vi "Сканер.vi"() -> ()   [LabVIEW 2016]
uses:
  GlobalVariable.vi
  <vilib>/Instr/_visa.llb/VISA Configure Serial Port (Instr).vi
panel:
  out "ReadNumber":i32
  out "Gauge":cluster{dbl, dbl}(knob) scale=0.0..360.0
  out "ScrollPosBool":bool
  out "Serial Settings:Number of Bytes at Serial Port":u32
  in  "XON/XOFF Символ":cluster{"XON":u8, "XOFF":u8}={"XON"=17, "XOFF"=19} {"XOFF" items=["NUL", "SOH", "STX", "ETX", "EOT", "ENQ", "ACK", "BEL", "BS", "HT", "LF", "VT", "FF", "CR", "SO", "SI", "DLE", "DC1", "DC2", "DC3", "DC4", "NAK", "SYN", "ETB", "CAN", "EM", "SUB", "ESC", "FS", "GS", "RS", "US", "SP", "!", "\"", "#", "$", "%", "&", "'", "(", ")", "*", "+", ",", "- (-)", ".", "/", "0", "1", "2", "3", "4", "5", "6", "7", "8", "9", ":", ";", "<", "=", ">", "?", "@", "A", "B", "C", "D", "E", "F", "G", "H", "I", "J", "K", "L", "M", "N", "O", "P", "Q", "R", "S", "T", "U", "V", "W", "X", "Y", "Z", "[", "\\", "]", "^", "_", "`", "a", "b", "c", "d", "e", "f", "g", "h", "i", "j", "k", "l", "m", "n", "o", "p", "q", "r", "s", "t", "u", "v", "w", "x", "y", "z", "{", "|", "}", "~"]; "XON" items=["NUL", "SOH", "STX", "ETX", "EOT", "ENQ", "ACK", "BEL", "BS", "HT", "LF", "VT", "FF", "CR", "SO", "SI", "DLE", "DC1", "DC2", "DC3", "DC4", "NAK", "SYN", "ETB", "CAN", "EM", "SUB", "ESC", "FS", "GS", "RS", "US", "SP", "!", "\"", "#", "$", "%", "&", "'", "(", ")", "*", "+", ",", "- (-)", ".", "/", "0", "1", "2", "3", "4", "5", "6", "7", "8", "9", ":", ";", "<", "=", ">", "?", "@", "A", "B", "C", "D", "E", "F", "G", "H", "I", "J", "K", "L", "M", "N", "O", "P", "Q", "R", "S", "T", "U", "V", "W", "X", "Y", "Z", "[", "\\", "]", "^", "_", "`", "a", "b", "c", "d", "e", "f", "g", "h", "i", "j", "k", "l", "m", "n", "o", "p", "q", "r", "s", "t", "u", "v", "w", "x", "y", "z", "{", "|", "}", "~"]}
  in  "Ошибка порта":T1
  in  "Номер COM порта":refnum<visa-resource-name>
  in  "Clear":bool
  in  "ReadStringON":bool
  in  "WriteStringON":bool
  in  "В конце записи добавить идентификатор завершения":bool=TRUE
  out "IndStartStop":bool
  in  "Exit":bool
  in  "Start":bool
  in  "Stop":bool
  out "Return Count Read":u32
  in  "В конце чтения добавить идентификатор завершения":bool=TRUE
  in  "Идентификатор завершения":u8=10 format="%.0x"
  out "Read String":string
  out "Return Count Write":u32
  in  "Write String":string="*IDN?"
  in  "Параметры порта":T2={"Бит в секунду: "=9600, "Биты данных:"=8, "Чётность"=0, "Стоповые биты"=10, "Управление потоком"=0} {"Управление потоком" items=["Нет"=0, "Xon/Xoff"=1, "RTS/CTS"=2, "DTR/DSR"=4]; "Стоповые биты" items=["1.0"=10, "1.5"=15, "2.0"=20]; "Чётность" items=["Нет", "Нечётный", "Чётный", "Маркер", "Пробел"]; "Биты данных:" items=["4"=4, "5"=5, "6"=6, "7"=7, "8"=8]; "Бит в секунду:" items=["75"=75, "110"=110, "134"=134, "150"=150, "300"=300, "600"=600, "1200"=1200, "1800"=1800, "2400"=2400, "4800"=4800, "7200"=7200, "9600"=9600, "14400"=14400, "19200"=19200, "28800"=28800, "38400"=38400, "56000"=56000, "57600"=57600, "115200"=115200, "128000"=128000, "230400"=230400]}
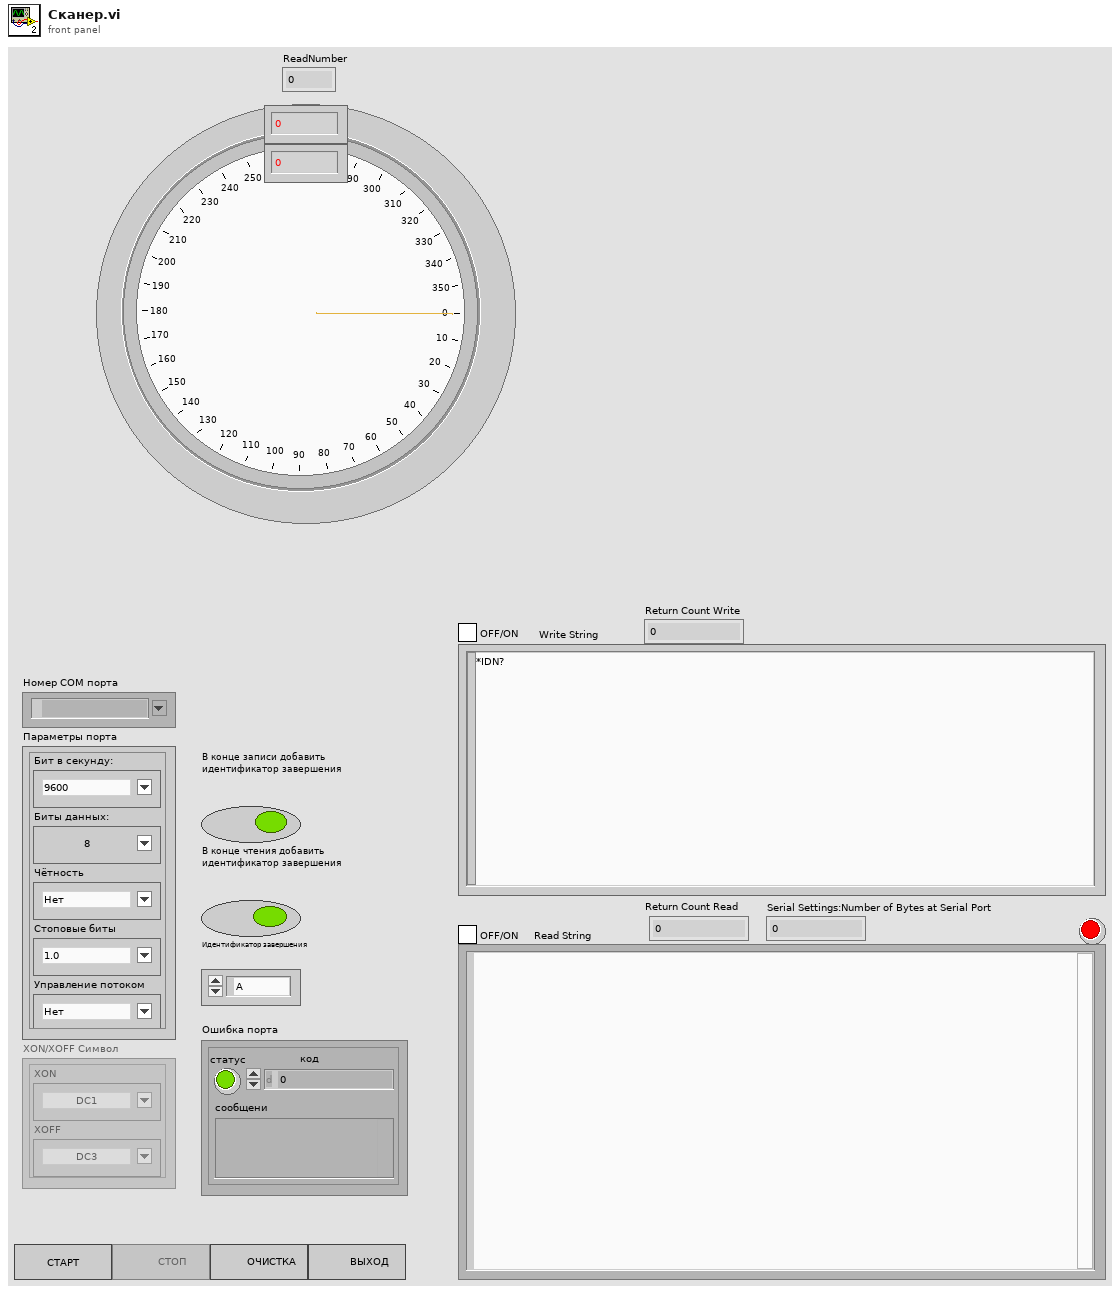
[diagram p1: front panel]
types:
  T1 = cluster{"статус":bool, "код":i32, "сообщени":string}
  T2 = cluster{"Бит в секунду: ":u32, "Биты данных:":u16, "Чётность":u16, "Стоповые биты":u16, "Управление потоком":u16}
  T3 = enum8{"Enabled", "Disabled", "Disabled and Grayed Out"}
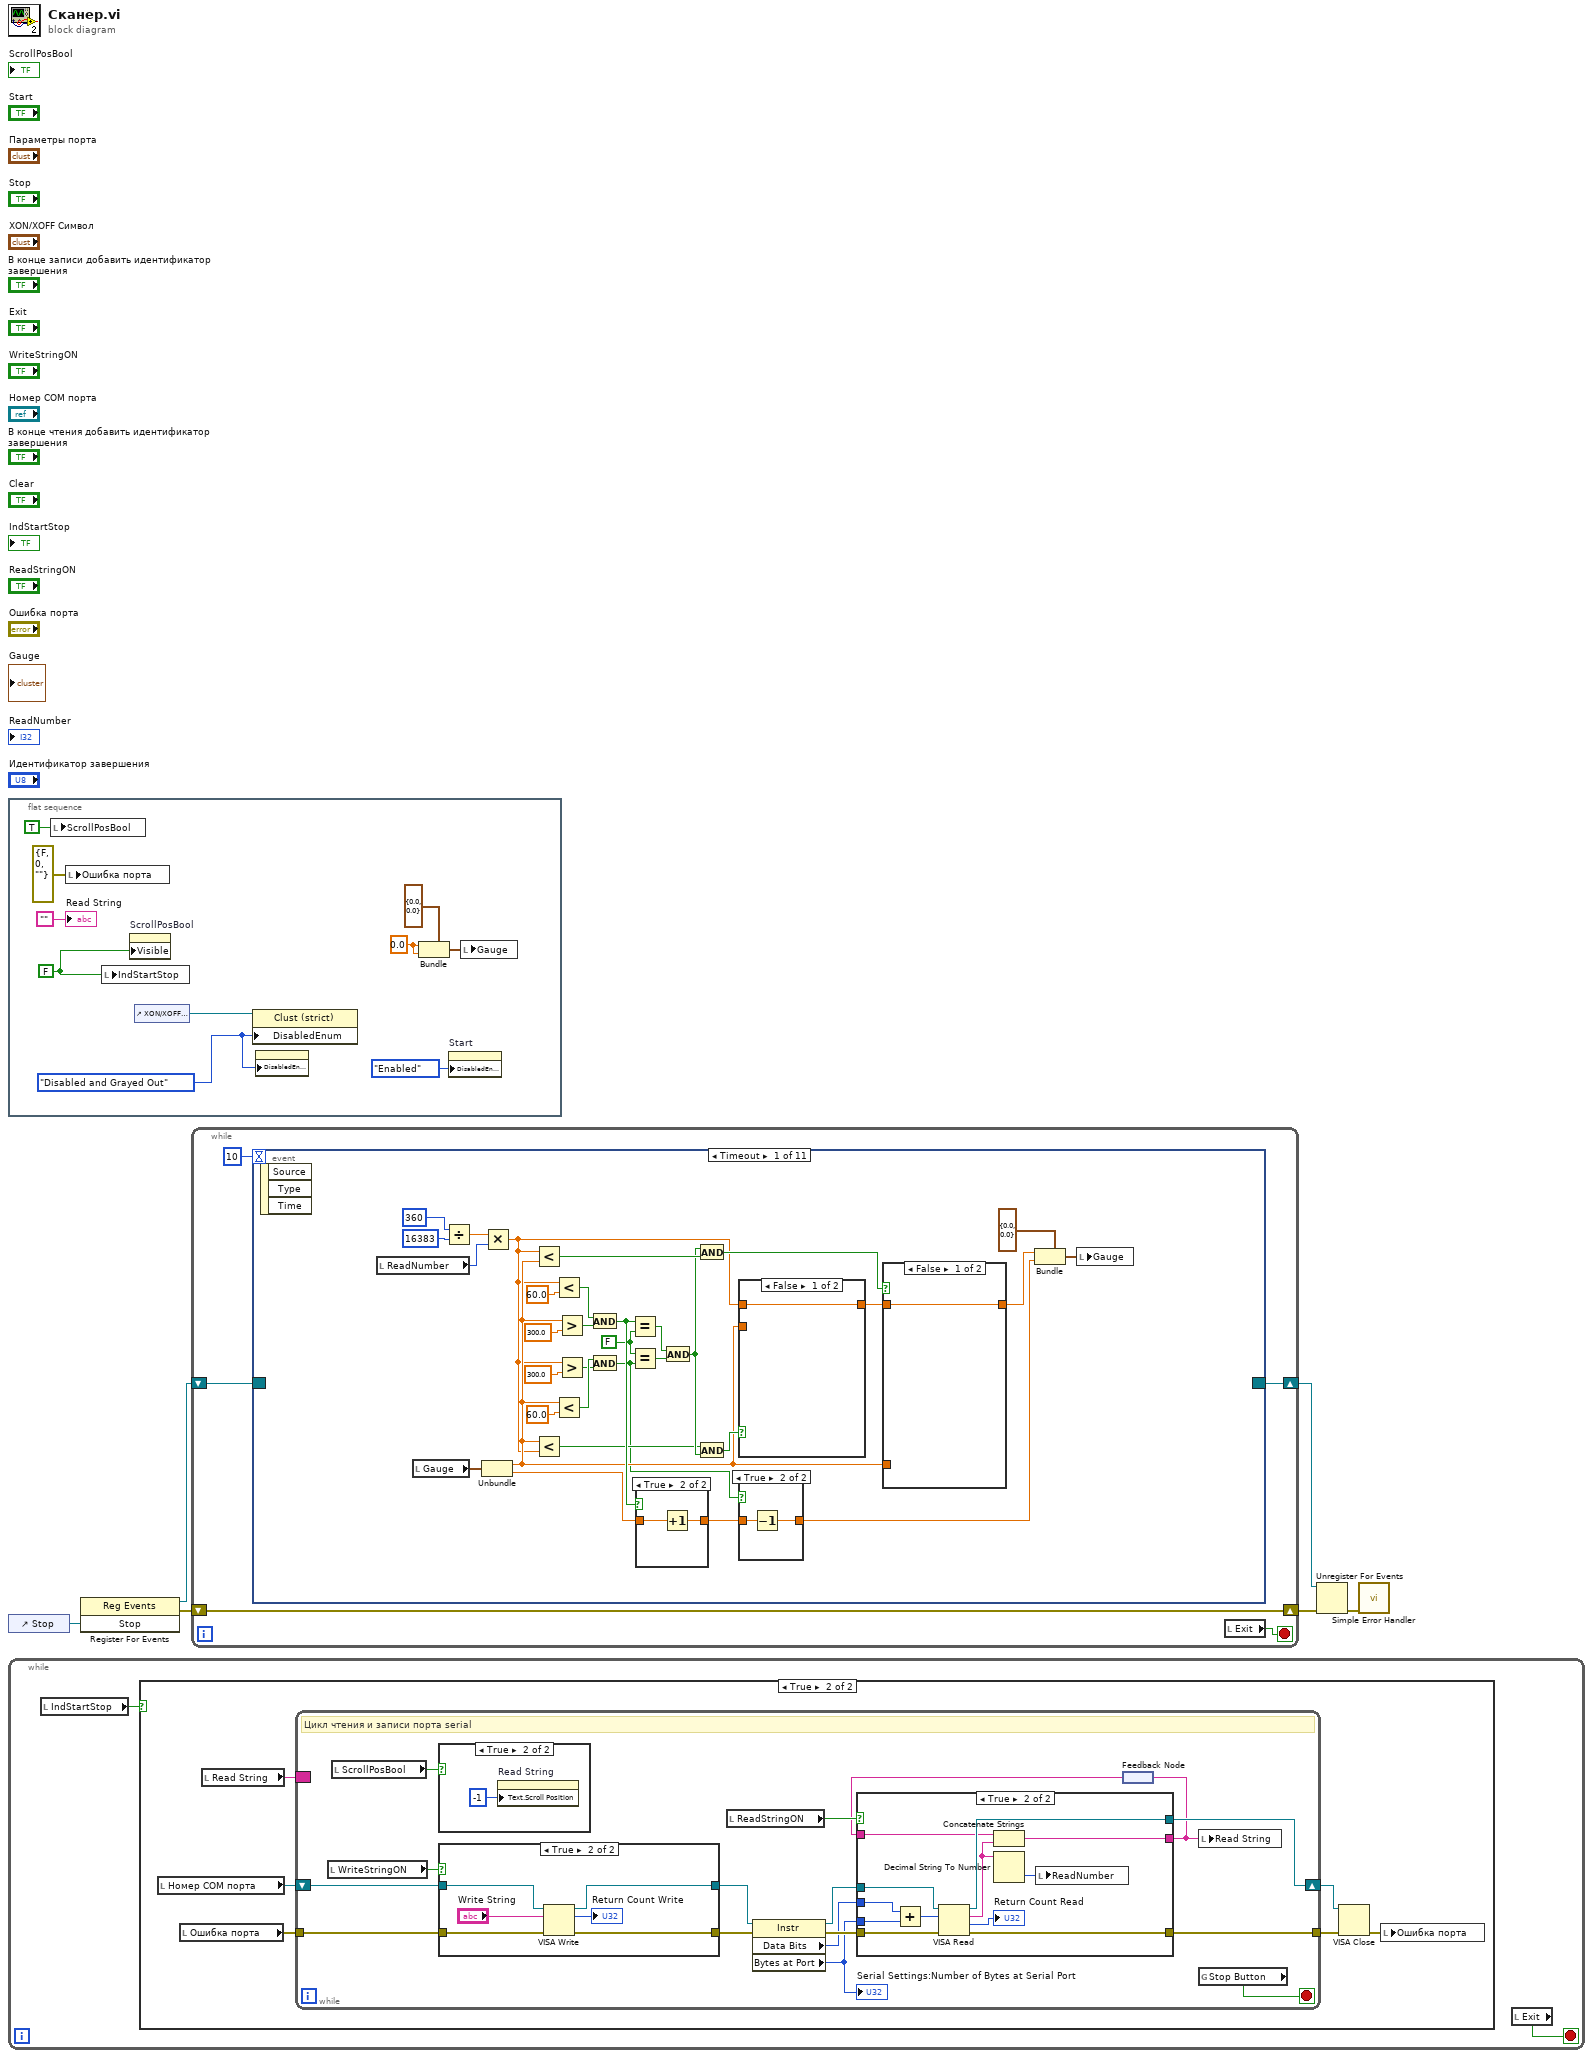
[diagram p0: block diagram]
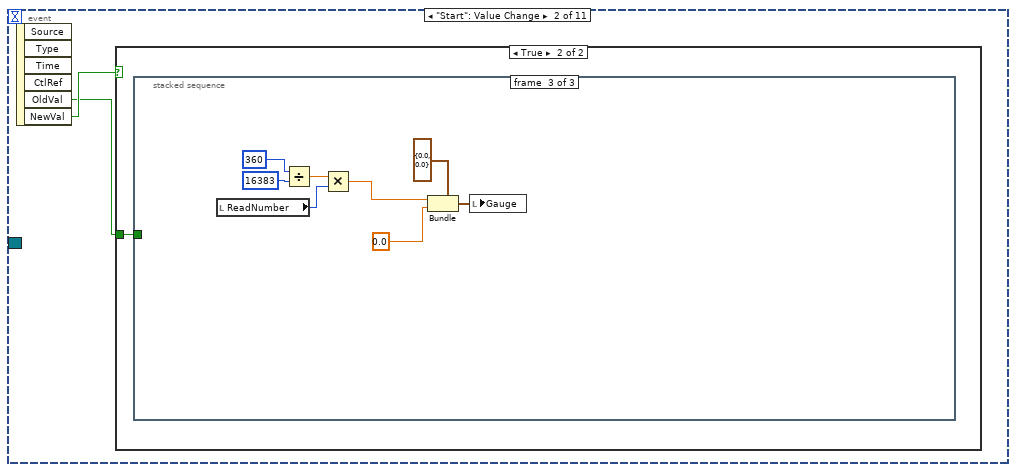
[diagram p10: hidden frame]
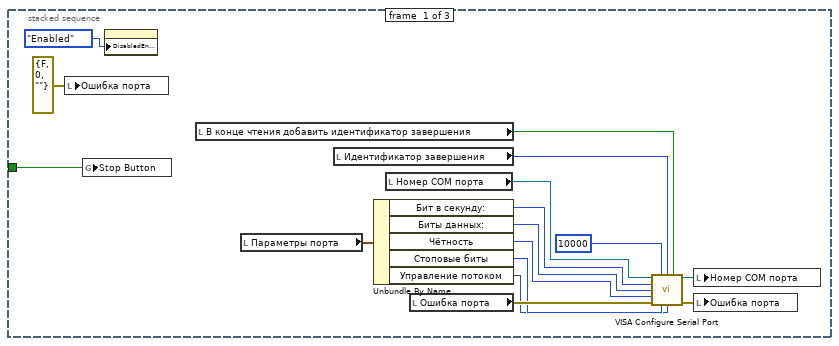
[diagram p12: hidden frame]
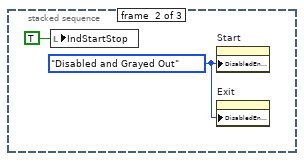
[diagram p13: hidden frame]
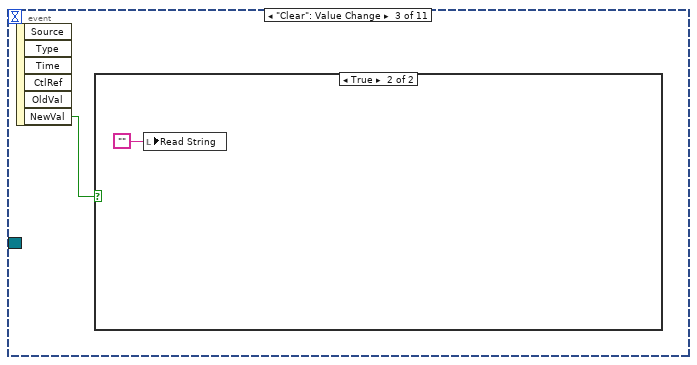
[diagram p14: hidden frame]
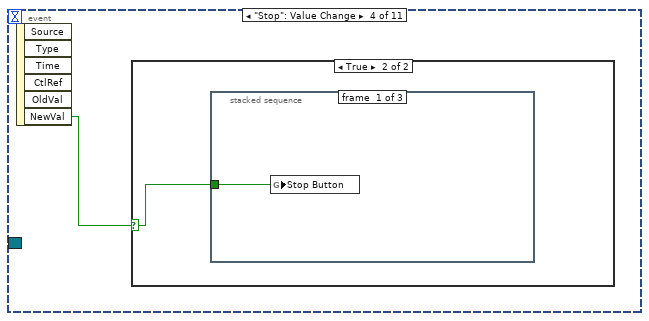
[diagram p16: hidden frame]
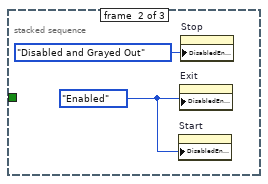
[diagram p18: hidden frame]
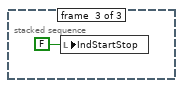
[diagram p19: hidden frame]
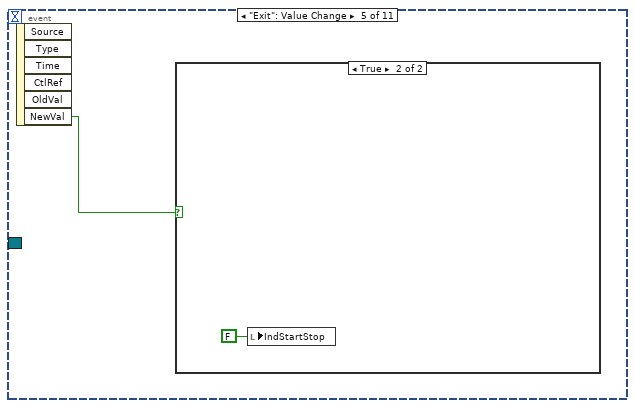
[diagram p20: hidden frame]
diagram:
  n1 = flat-sequence {
    frame #0 {
      w7 = 0.0
      w12 = FALSE
      w11 = T3."Disabled and Grayed Out" ("Disabled")
      n2 = local write "ScrollPosBool"(TRUE ("ScrollPosBool")) -> ()
      n3 = local write "Ошибка порта"(errorcluster {"status"=FALSE, "code"=0, "source"=""} ("error in (no error)")) -> ()
      n4 = local write "IndStartStop"(w12) -> ()
      n5 = property on="ScrollPosBool" class="Bool (strict)"("Visible"=w12) -> ()  [unwired: 2 in, 2 out]
      n6 = control-ref of="XON/XOFF Символ"() -> (w15:refnum<vi>)
      n7 = property class="Clust (strict)"(reference=w15, "DisabledEnum"=w11) -> ()  [unwired: 1 in, 2 out]
      n8 = property on="Stop" class="Bool (strict)"("DisabledEnum"=w11) -> ()  [unwired: 2 in, 2 out]
      n9 = Bundle(cluster=cluster{dbl, dbl} {0.0, 0.0} ("Gauge"), w7, w7) -> (w9:cluster{dbl, dbl})
      n10 = property on="Start" class="Bool (strict)"("DisabledEnum"=T3."Enabled" ("Disabled")) -> ()  [unwired: 2 in, 2 out]
      n11 = local write "Gauge"(w9) -> ()
      "Read String" <- ""
    }
  }
  n12 = control-ref of="Stop"() -> (w1:refnum<vi>)
  n13 = while {
    stop <- w17 stop-if-true
    n14 = local read "IndStartStop"() -> (w18:bool)
    n15 = case shown="True" w18 {
      frame False {
      }
      frame True {
        n16 = local read "Номер COM порта"() -> (w23:refnum<visa-resource-name>)
        n17 = local read "Ошибка порта"() -> (w24:T1)
        n18 = local read "Read String"() -> (w22:string)
        n19 = while {
          shift-right: [w31] -> w20
          shift-left: w23 -> [w32]
          tunnel: w24 -> [w33]
          tunnel: [w30] -> w19
          border: w22 -> [_]
          stop <- w27 stop-if-true
          # "Цикл чтения и записи порта serial"
          n20 = local read "WriteStringON"() -> (w36:bool)
          n21 = local read "ScrollPosBool"() -> (w34:bool)
          n22 = case shown="True" w34 {
            frame False {
            }
            frame True {
              n23 = property on="Read String" class="Str"("Text.Scroll Position"=-1) -> ()  [unwired: 2 in, 2 out]
            }
          }
          n24 = case shown="True" w36 {
            tunnel: [w58 w64] -> w40
            tunnel: [w57 w63] -> w39
            tunnel: w32 -> [w58 w62]
            tunnel: w33 -> [w57 w61]
            frame False {
            }
            frame True {
              n25 = VISA Write(VISA resource name=w62, write buffer="Write String", error in (no error)=w61) -> (VISA resource name out=w64:refnum<visa-resource-name>, return count=→"Return Count Write":u32, error out=w63:errorcluster)
            }
          }
          n26 = local read "ReadStringON"() -> (w35:bool)
          n27 = property class="Instr"(reference=w40, error in=w39) -> (reference out=w38:refnum<visa-resource-name>, error out=w37:errorcluster, "Data Bits"=w26:u16, "Bytes at Port"=w25:u32)
          "Serial Settings:Number of Bytes at Serial Port" <- w25
          n28 = feedback #1() -> (w29:string)
          n29 = case shown="True" w35 {
            tunnel: [w44 w56] -> w31
            tunnel: [w43 w52] -> w30
            tunnel: w25 -> [_ w51]
            tunnel: w38 -> [w44 w55]
            tunnel: w37 -> [w43 w54]
            tunnel: [w42 w49] -> w28
            tunnel: w29 -> [w42 w48]
            tunnel: w26 -> [_ w47]
            frame False {
            }
            frame True {
              n30 = Add(x=w47, y=w51) -> (x+y=w50:u32)
              n31 = VISA Read(VISA resource name=w55, byte count=w50, error in (no error)=w54) -> (VISA resource name out=w56:refnum<visa-resource-name>, read buffer=w46:string, return count=→"Return Count Read":u32, error out=w52:errorcluster)
              n32 = Concatenate Strings(w48, w46) -> (w49:string)
              n33 = Decimal String To Number(string=w46) -> (number=w45:i32)  [unwired: 2 in, 1 out]
              n34 = local write "ReadNumber"(w45) -> ()
            }
          }
          n35 = feedback-in #1(w28) -> ()
          n36 = local write "Read String"(w28) -> ()
          n37 = global read "GlobalVariable.vi" "Stop Button"() -> (w27:bool)
        }
        n38 = VISA Close(VISA resource name=w20, error in (no error)=w19) -> (error out=w21:errorcluster)
        n39 = local write "Ошибка порта"(w21) -> ()
      }
    }
    n40 = local read "Exit"() -> (w17:bool)
  }
  n41 = register-events(w1) -> (reference out=w6:refnum<event-registration>, error out=w5:errorcluster)  [unwired: 2 in]
  n42 = while {
    shift-right: [w67] -> w4
    shift-left: w6 -> [w68]
    shift-right: [w66] -> w3
    shift-left: w5 -> [w66]
    stop <- w65 stop-if-true
    n43 = event shown="[0] Timeout" {
      selector: w68 -> [_ _ _ _ _ _ _ _ _ _ _]
      dyn-events: [_ _ _ _ _ _ _ _ _ _ _] -> w67
      timeout: 10 -> [_ _ _ _ _ _ _ _ _ _ _]
      event Timeout {
        w72 = FALSE
        n44 = event-data() -> ()  [unwired: 1 in, 3 out]
        n45 = local read "ReadNumber"() -> (w100:i32)
        n46 = local read "Gauge"() -> (w96:cluster{dbl, dbl})
        n47 = Divide(x=360 ("y"), y=16383 ("x")) -> (x/y=w101:dbl)
        n48 = Unbundle(w96) -> (w75:dbl, w86:dbl)
        n49 = Multiply(x=w101, y=w100) -> (x*y=w70:dbl)
        n50 = Less?(x=w70, y=w75) -> (x < y?=w79:bool)
        n51 = Less?(x=w75, y=w70) -> (x < y?=w73:bool)
        n52 = Less?(x=w70, y=60.0) -> (x < y?=w92:bool)
        n53 = Less?(x=w75, y=60.0) -> (x < y?=w88:bool)
        n54 = Greater?(x=w75, y=300.0) -> (0:w91:bool)
        n55 = Greater?(x=w70, y=300.0) -> (0:w87:bool)
        n56 = And(x=w92, y=w91) -> (x .and. y?=w80:bool)
        n57 = And(x=w88, y=w87) -> (x .and. y?=w71:bool)
        n58 = Equal?(x=w80, y=w72) -> (x = y?=w84:bool)
        n59 = Equal?(x=w72, y=w71) -> (x = y?=w83:bool)
        n60 = case shown="True" w80 {
          tunnel: w86 -> [w109 w111]
          tunnel: [w109 w110] -> w85
          frame False {
          }
          frame True {
            n61 = Increment(x=w111) -> (x+1=w110:dbl)
          }
        }
        n62 = And(x=w84, y=w83) -> (x .and. y?=w74:bool)
        n63 = And(x=w74, y=w79) -> (x .and. y?=w78:bool)
        n64 = And(x=w73, y=w74) -> (x .and. y?=w82:bool)
        n65 = case shown="False" w82 {
          tunnel: w70 -> [w104 w105]
          tunnel: w75 -> [_ _]
          tunnel: [w104 w105] -> w77
          frame False {
          }
          frame True {
          }
        }
        n66 = case shown="True" w71 {
          tunnel: w85 -> [w106 w108]
          tunnel: [w106 w107] -> w81
          frame False {
          }
          frame True {
            n67 = Decrement(x=w108) -> (x-1=w107:dbl)
          }
        }
        n68 = case shown="False" w78 {
          tunnel: [w102 w103] -> w76
          tunnel: w75 -> [_ _]
          tunnel: w77 -> [w102 w103]
          frame False {
          }
          frame True {
          }
        }
        n69 = Bundle(cluster=cluster{dbl, dbl} {0.0, 0.0} ("Gauge"), w76, w81) -> (w97:cluster{dbl, dbl})
        n70 = local write "Gauge"(w97) -> ()
      }
      event "Start": Value Change {
        n71 = event-data() -> ("OldVal"=w112:bool, "NewVal"=w113:bool)  [unwired: 1 in, 4 out]
        n72 = case shown="True" w113 {
          tunnel: w112 -> [_ w114]
          frame False {
          }
          frame True {
            n73 = stacked-sequence {
              tunnel: w114 -> [w115 _ _]
              frame #0 {
                n74 = local write "Ошибка порта"(errorcluster {"status"=FALSE, "code"=0, "source"=""} ("error in (no error)")) -> ()
                n75 = global write "GlobalVariable.vi" "Stop Button"(w115) -> ()
                n76 = property on="Stop" class="Bool (strict)"("DisabledEnum"=T3."Enabled" ("Disabled")) -> ()  [unwired: 2 in, 2 out]
                n77 = local read "В конце чтения добавить идентификатор завершения"() -> (w128:bool)
                n78 = local read "Параметры порта"() -> (w124:T2)
                n79 = local read "Идентификатор завершения"() -> (w127:u8)
                n80 = Unbundle By Name(w124) -> ("Бит в секунду:"=w123:u32, "Биты данных:"=w122:u16, "Чётность"=w121:u16, "Стоповые биты"=w120:u16, "Управление потоком"=w119:u16)
                n81 = local read "Номер COM порта"() -> (w125:refnum<visa-resource-name>)
                n82 = local read "Ошибка порта"() -> (w126:T1)
                n83 = call-poly "VISA Configure Serial Port"("VISA resource name"=w125, "timeout (10sec)"=u32 10000, "termination char\n(0xA = '\\n' = LF)"=w127, "Enable Termination\nChar (T)"=w128, "baud rate (9600)"=w123, "data bits (8)"=w122, "parity (0:none)"=w121, "error in (no error)"=w126, "stop bits (10: 1 bit)"=w120, "flow control (0:none)"=w119) -> ("VISA resource name out"=w117:refnum<visa-resource-name>, "error out"=w116:errorcluster)  [unwired: 4 in]
                n84 = local write "Номер COM порта"(w117) -> ()
                n85 = local write "Ошибка порта"(w116) -> ()
              }
              frame #1 {
                w131 = T3."Disabled and Grayed Out" ("Disabled")
                n86 = local write "IndStartStop"(TRUE) -> ()
                n87 = property on="Start" class="Bool (strict)"("DisabledEnum"=w131) -> ()  [unwired: 2 in, 2 out]
                n88 = property on="Exit" class="Bool (strict)"("DisabledEnum"=w131) -> ()  [unwired: 2 in, 2 out]
              }
              frame #2 {
                n89 = local read "ReadNumber"() -> (w136:i32)
                n90 = Divide(x=360 ("y"), y=16383 ("x")) -> (x/y=w137:dbl)
                n91 = Multiply(x=w137, y=w136) -> (x*y=w133:dbl)
                n92 = Bundle(cluster=cluster{dbl, dbl} {0.0, 0.0} ("Gauge"), w133, 0.0) -> (w138:cluster{dbl, dbl})
                n93 = local write "Gauge"(w138) -> ()
              }
            }
          }
        }
      }
      event "Clear": Value Change {
        n94 = event-data() -> ("NewVal"=w141:bool)  [unwired: 1 in, 5 out]
        n95 = case shown="True" w141 {
          frame False {
          }
          frame True {
            n96 = local write "Read String"("") -> ()
          }
        }
      }
      event "Stop": Value Change {
        n97 = event-data() -> ("NewVal"=w143:bool)  [unwired: 1 in, 5 out]
        n98 = case shown="True" w143 {
          selector: w143 -> [_ w144]
          frame False {
          }
          frame True {
            n99 = stacked-sequence {
              tunnel: w144 -> [w145 _ _]
              frame #0 {
                n100 = global write "GlobalVariable.vi" "Stop Button"(w145) -> ()
              }
              frame #1 {
                w147 = T3."Enabled" ("Disabled")
                n101 = property on="Start" class="Bool (strict)"("DisabledEnum"=w147) -> ()  [unwired: 2 in, 2 out]
                n102 = property on="Exit" class="Bool (strict)"("DisabledEnum"=w147) -> ()  [unwired: 2 in, 2 out]
                n103 = property on="Stop" class="Bool (strict)"("DisabledEnum"=T3."Disabled and Grayed Out" ("Disabled")) -> ()  [unwired: 2 in, 2 out]
              }
              frame #2 {
                n104 = local write "IndStartStop"(FALSE) -> ()
              }
            }
          }
        }
      }
      event "Exit": Value Change {
        n105 = event-data() -> ("NewVal"=w149:bool)  [unwired: 1 in, 5 out]
        n106 = case shown="True" w149 {
          frame False {
          }
          frame True {
            n107 = local write "IndStartStop"(FALSE) -> ()
          }
        }
      }
      event "Параметры порта.Управление потоком": Value Change {
        n108 = event-data() -> ("NewVal"=w151:u16)  [unwired: 1 in, 5 out]
        n109 = case shown="1" w151 {
          frame Default {
            n110 = control-ref of="XON/XOFF Символ"() -> (w152:refnum<vi>)
            n111 = property class="Clust (strict)"(reference=w152, "DisabledEnum"=T3."Disabled and Grayed Out" ("Disabled")) -> ()  [unwired: 1 in, 2 out]
          }
          frame 1 {
            n112 = control-ref of="XON/XOFF Символ"() -> (w154:refnum<vi>)
            n113 = property class="Clust (strict)"(reference=w154, "DisabledEnum"=T3."Enabled" ("Disabled")) -> ()  [unwired: 1 in, 2 out]
          }
        }
      }
      event "Параметры порта": Value Change {
        n114 = event-data() -> ("NewVal"=w165:T2)  [unwired: 1 in, 5 out]
        n115 = Unbundle By Name(w165) -> ("Бит в секунду:"=w160:u32, "Биты данных:"=w159:u16, "Чётность"=w158:u16, "Стоповые биты"=w157:u16, "Управление потоком"=w156:u16)
        n116 = local read "Номер COM порта"() -> (w164:refnum<visa-resource-name>)
        n117 = local read "Ошибка порта"() -> (w163:T1)
        n118 = property class="Instr"(reference=w164, error in=w163, "Baud"=w160, "Data Bits"=w159, "Parity"=w158, "Stop Bits"=w157, "Flow Cntrl"=w156) -> (reference out=w162:refnum<visa-resource-name>, error out=w161:errorcluster)
        n119 = local write "Номер COM порта"(w162) -> ()
        n120 = local write "Ошибка порта"(w161) -> ()
      }
      event "Номер COM порта": Value Change {
        n121 = event-data() -> ("NewVal"=w166:refnum<visa-resource-name>)  [unwired: 1 in, 5 out]
        n122 = local write "Номер COM порта"(w166) -> ()
      }
      event "XON/XOFF Символ": Value Change {
        n123 = event-data() -> ("NewVal"=w169:cluster{"XON":u8, "XOFF":u8})  [unwired: 1 in, 5 out]
        n124 = local read "Номер COM порта"() -> (w171:refnum<visa-resource-name>)
        n125 = Unbundle(w169) -> ("XON"=w168:u8, "XOFF"=w167:u8)
        n126 = property class="Instr"(reference=w171, "XON Char"=w168, "XOFF Char"=w167) -> (reference out=w170:refnum<visa-resource-name>)  [unwired: 1 in, 1 out]
        n127 = local write "Номер COM порта"(w170) -> ()
      }
      event "В конце записи добавить идентификатор завершения": Value Change {
        n128 = event-data() -> ("NewVal"=w176:bool)  [unwired: 1 in, 5 out]
        n129 = local read "Идентификатор завершения"() -> (w177:u8)
        n130 = local read "Номер COM порта"() -> (w175:refnum<visa-resource-name>)
        n131 = local read "Ошибка порта"() -> (w173:T1)
        n132 = case shown="True" w176 {
          tunnel: w177 -> [_ w184]
          tunnel: w175 -> [w179 w183]
          tunnel: [w179 w182] -> w174
          tunnel: w173 -> [w178 w181]
          tunnel: [w178 w180] -> w172
          frame False {
          }
          frame True {
            w186 = u16 2 items=["None", "LastBit", "TermChar", "Break"] ("Serial Settings:Serial End Mode for Writes")
            n133 = property class="Instr"(reference=w183, error in=w181, "Serial Settings:End Mode for Writes"=w186, "Message Based Settings:Send End Enable"=TRUE, "Message Based Settings:Termination Character"=w184) -> (reference out=w182:refnum<visa-resource-name>, error out=w180:errorcluster)
          }
        }
        n134 = local write "Номер COM порта"(w174) -> ()
        n135 = local write "Ошибка порта"(w172) -> ()
      }
      event "Read String": Shortcut Menu Selection (User) {
        n136 = event-data() -> ("ItemTag"=w187:string)  [unwired: 1 in, 7 out]
        n137 = case shown="\"USER_MENU_ITEM_2\"" w187 {
          frame "USER_MENU_ITEM_1" {
            n138 = local write "ScrollPosBool"(TRUE ("ScrollPosBool")) -> ()
          }
          frame Default {
          }
          frame "USER_MENU_ITEM_2" {
            n139 = local write "ScrollPosBool"(FALSE ("ScrollPosBool")) -> ()
          }
        }
      }
    }
    n140 = local read "Exit"() -> (w65:bool)
  }
  n141 = Unregister For Events(event registration refnum=w4, error in=w3) -> (error out=w2:errorcluster)
  n142 = call <vilib>:"Simple Error Handler.vi"("error in (no error)"=w2) -> ()  [unwired: 4 in, 5 out]
